vi "Z6_Beamline.color Northtower BL.vi"(0 "i ref in":refnum<vi>, 2 "Color State Northtower Input":i32, 5 "error in (no error)":errorcluster) -> (14 "i ref out":refnum<vi>, 16 "Color State Northwower Exit":i32, 19 "error out":errorcluster)   [LabVIEW 2014, in "Z6_Beamline.lvlib"]
doc: "This Vi colors the Mirrortower beamline elements."
uses:
  Z6_Beamline.lvlib
  PH_Basics/PH_Common/PH_Common.lvlib
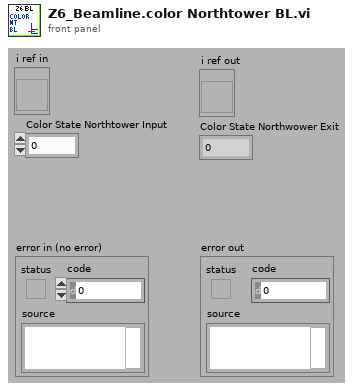
[diagram p1: front panel]
types:
  T1 = typedef "Z6_Beamline.lvlib/Z6_Beamline.i attribute.ctl" = cluster{"Subs ok GUI Refs":T2, "Refs BL Northtower":refnum<vi>[], "Refs BL Southtower":refnum<vi>[], "Refs BL 100TW COS":refnum<vi>[], "State Subsystems":cluster{"Northtower":bool, "Southtower":bool, "Frontends":bool, "100TW COS":bool}, "Z6 Beamline Status Subscriber Information":T3, "Color State PHELIX":i16}
  T2 = typedef "Z6_Beamline.lvlib/Z6_Beamline.Subsystem ok GUI Refs.ctl" = cluster{"Northtower ok":refnum<vi>, "Southtower ok":refnum<vi>, "Frontends ok":refnum<vi>, "100TW COS ok":refnum<vi>}
  T3 = typedef "Z6_Beamline.lvlib/Z6_Beamline.Status Subscriber Information.ctl" = cluster{"BL Z6 Shutter":T4, "CH 10":T4, "CH 11":T4, "ST Flip Cam":T4, "ST Flip DB":T4, "BL Z6 Dump":T4}
  T4 = typedef "PH_BL-Master.lvlib/PH_BL-Master.Status Subscriber Information.ctl" = cluster{"Index of element":i32, "Attributeset":T5}
  T5 = typedef "PH_BL-Master.lvlib/PH_BL-Master.Attribute Set.ctl" = enum16{"Boolean Status Service Subscriber", "Picture Status Service Subscriber"}
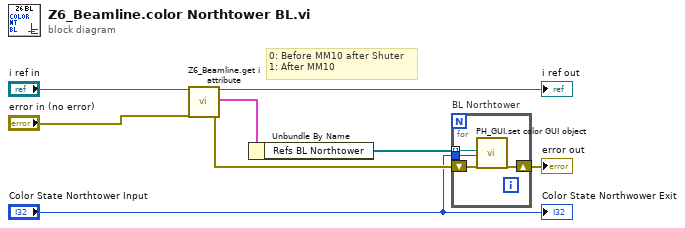
[diagram p0: block diagram]
diagram:
  # "0: Before MM10 after Shuter\n1: After MM10"
  n1 = call "Z6_Beamline.get i attribute.vi"("i ref in"="i ref in", "error in (no error)"="error in (no error)") -> ("i ref out"=→"i ref out":refnum<vi>, "i attribute"=w8:T1, "error out"=w5:errorcluster)  [unwired: 15 in]
  n2 = Unbundle By Name(w8) -> ("Refs BL Northtower"=w6:refnum<vi>[])
  n3 = for "BL Northtower" {
    tunnel: w6 -> [w12] mode=indexing
    shift-right: [w10] -> w4
    shift-left: w5 -> [w11]
    tunnel: "Color State Northtower Input" -> [w9]
    n4 = call "PH_GUI.set color GUI object.vi"("GUI object Ref"=w12, "State"=w9, "error in (no error)"=w11) -> ("error out"=w10:errorcluster)  [unwired: 16 in]
  }
  "error out" <- w4
  "Color State Northwower Exit" <- "Color State Northtower Input"
